vi "XGT 연속쓰기 Enquire.vi"(5 "명령어타입":string="SB", 6 "BCC":string, 7 "명령어":string="W", 8 "데이터개수":string="01", 9 "변수이름":string="%DW000", 10 "변수길이":string="06", 11 "국번":string="01") -> (2 "연속연결 Enquire문":string)   [LabVIEW 2012]
panel:
  in  "데이터":string[](array[string])=["AA15"]
  in  "Header":string="\u0005"
  in  "Tail":string="\u0004"
  # "변수 이름=시작주소를 의미함."
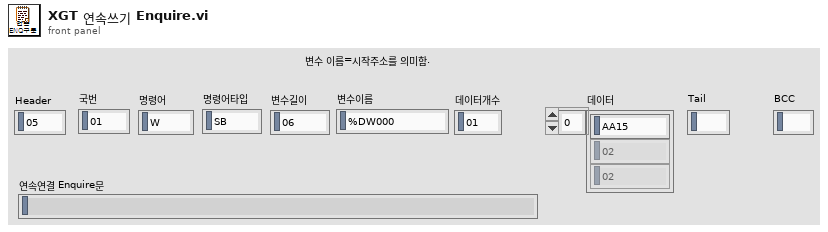
[diagram p1: front panel]
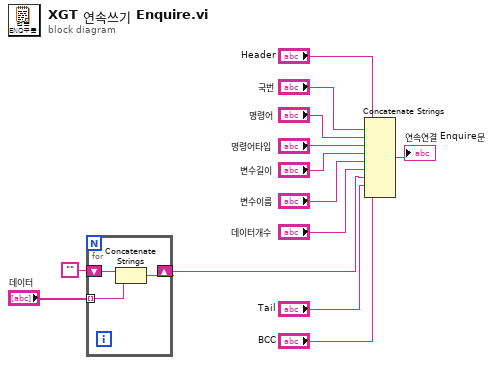
[diagram p0: block diagram]
diagram:
  n1 = for {
    tunnel: "데이터" -> [w15] mode=indexing
    shift-right: [w14] -> w3
    shift-left: "" -> [w16]
    n2 = Concatenate Strings(w16, w15) -> (w14:string)
  }
  n3 = Concatenate Strings("Header", "국번", "명령어", "명령어타입", "변수길이", "변수이름", "데이터개수", w3, "Tail", "BCC") -> (→"연속연결 Enquire문":string)
